vi "Simulation Finalize.vi"(6 "terminated by user?":bool, 8 "error in (no error)":errorcluster, 11 "simulator":T1={"configuration"={"maxTime"=5.0, "enableVisualization"=TRUE, "statechart"=path "iRobot Navigation State Machine.vi", "environment"=path "simulation configuration.ini", "record"=path "Simulation Record.xml", "autograde?"=TRUE, "interactive?"=FALSE, "feedback mode"=enum."debug navigation"}, "Bump Sensors"=[], "Distance Sensors"=[], "Accelerometer"=refnum, "Wall Sensor"=refnum, "Statechart\ndisplay"=refnum, "Body"=refnum, "Left Motor"=refnum, "Right Motor"=refnum, "first step?"=FALSE}) -> (0 "error out":errorcluster, 3 "simulator":T1={"configuration"={"maxTime"=5.0, "enableVisualization"=TRUE, "statechart"=path "iRobot Navigation State Machine.vi", "environment"=path "simulation configuration.ini", "record"=path "Simulation Record.xml", "autograde?"=TRUE, "interactive?"=FALSE, "feedback mode"=enum."debug navigation"}, "Bump Sensors"=[], "Distance Sensors"=[], "Accelerometer"=refnum, "Wall Sensor"=refnum, "Statechart\ndisplay"=refnum, "Body"=refnum, "Left Motor"=refnum, "Right Motor"=refnum, "first step?"=FALSE})   [LabVIEW 2013]
uses:
  Simulator.ctl
  <instrlib>/DC Motor Controller/HAIOL/DC Motor Controller.lvclass
  CyberSim interface/Simulation Configuration.ctl
  autograder/feedbackMode.ctl
  Simulation Call Statechart Operation.ctl
  <vilib>/robotics/Simulator/NI_Robotics_Simulator.lvlib
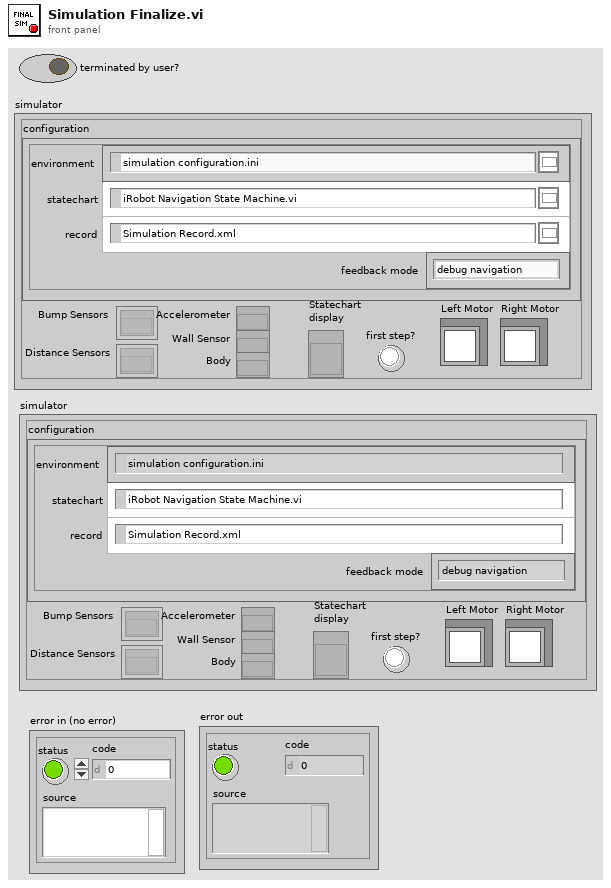
[diagram p1: front panel]
types:
  T1 = typedef "Simulator.ctl" = cluster{"configuration":T2, "Bump Sensors":refnum<k20>[], "Distance Sensors":refnum<k20>[], "Accelerometer":refnum<k20>, "Wall Sensor":refnum<k20>, "Statechart\ndisplay":refnum<vi>, "Body":refnum<k20>, "Left Motor":refnum<class "DC Motor Controller.lvclass">, "Right Motor":refnum<class "DC Motor Controller.lvclass">, "first step?":bool}
  T2 = typedef "Simulation Configuration.ctl" = cluster{"maxTime":sgl, "enableVisualization":bool, "statechart":path, "environment":path, "record":path, "autograde?":bool, "interactive?":bool, "feedback mode":T3}
  T3 = typedef "feedbackMode.ctl" = enum32{"debug navigation", "debug hill climb", "autograde navigation", "autograde hill climb"}
  T4 = typedef "Simulation Call Statechart Operation.ctl" = enum16{"Initialize", "Call Statechart", "Finalize"}
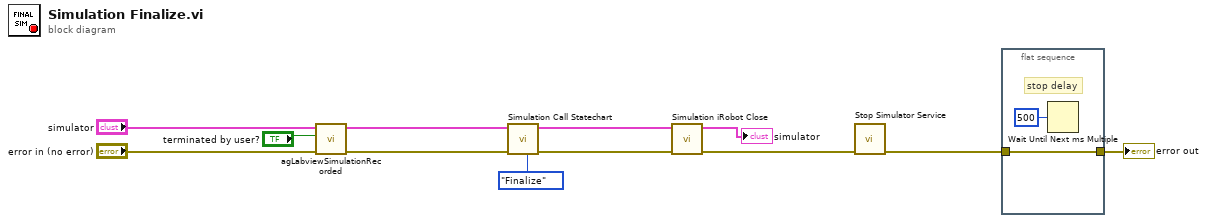
[diagram p0: block diagram]
diagram:
  n1 = call "agLabviewSimulationRecorded.vi"("Error In"="error in (no error)", "terminated by user?"="terminated by user?", "simulator"="simulator") -> ("Error Out"=w7:errorcluster, "simulator"=w6:T1)  [unwired: 7 in]
  n2 = call "Simulation Call Statechart.vi"("operation"=Simulation_Call_Statechart_Operation."Finalize", "error in"=w7, "simulator"=w6) -> ("error out"=w10:errorcluster, "simulator"=w11:T1)  [unwired: 6 in, 1 out]
  n3 = call "Simulation iRobot Close.vi"("error in"=w10, "simulator"=w11) -> ("error out"=w12:errorcluster, "simulator"=→"simulator":T1)  [unwired: 8 in]
  n4 = call <vilib>:"Stop Simulator Service.vi"("error in (no error)"=w12) -> ("error out"=w5:errorcluster)  [unwired: 10 in]
  n5 = flat-sequence {
    tunnel: w5 -> [w14]
    tunnel: [w14] -> w4
    frame #0 {
      # "stop delay"
      n6 = Wait Until Next ms Multiple(millisecond multiple=u32 500) -> ()  [unwired: 1 out]
    }
  }
  "error out" <- w4
